vi "TranslateTyping.vi"(11 "Cluster":T2) -> (3 "string":string)   [LabVIEW 2016]
uses:
  <vilib>/event_ctls.llb/eventvkey.ctl
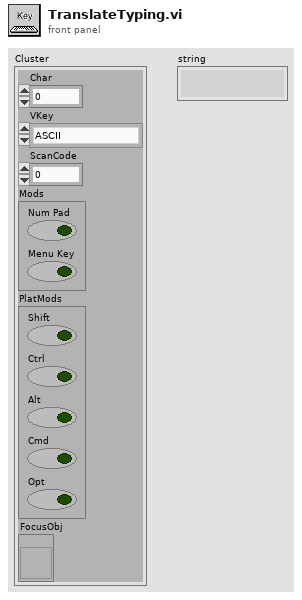
[diagram p1: front panel]
types:
  T1 = typedef "eventvkey.ctl" = enum16{"ASCII", "Enter", "Return", "Shift", "Ctrl", "Alt", "Cmd", "Opt", "Caps", "NumLock", "Clear", "Break", "Up", "Down", "Left", "Right", "Insert", "Delete", "Home", "End", "PageUp", "PageDown", "Escape", "Help", "Pause", "ScrollLock", "F1", "F2", "F3", "F4", "F5", "F6", "F7", "F8", "F9", "F10", "F11", "F12", "F13", "F14", "F15", "F16", "F17", "F18", "F19", "F20", "F21", "F22", "F23", "F24", "Play", "VolumeUp", "VolumeDown", "Mute", "Two Byte Char"}
  T2 = cluster{"Char":i16, "VKey":T1, "ScanCode":i16, "Mods":cluster{"Num Pad":bool, "Menu Key":bool}, "PlatMods":cluster{"Shift":bool, "Ctrl":bool, "Alt":bool, "Cmd":bool, "Opt":bool}, "FocusObj":refnum<vi>}
  T3 = cluster{"Shift":bool, "Ctrl":bool, "Alt":bool, "Cmd":bool, "Opt":bool}
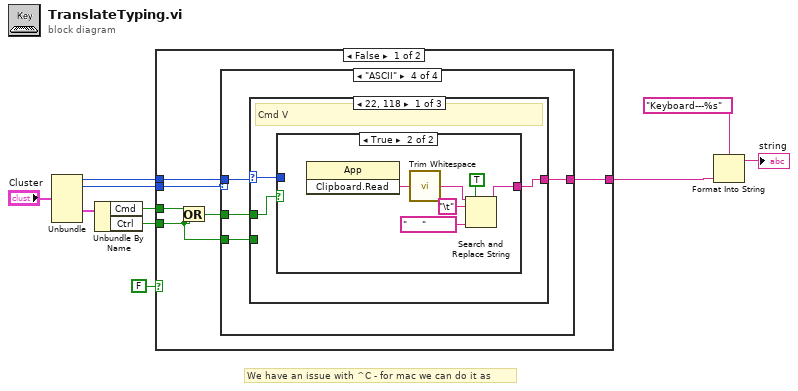
[diagram p0: block diagram]
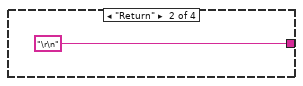
[diagram p3: hidden frame]
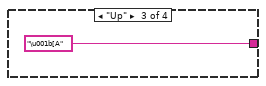
[diagram p4: hidden frame]
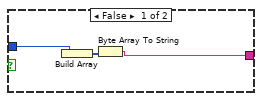
[diagram p5: hidden frame]
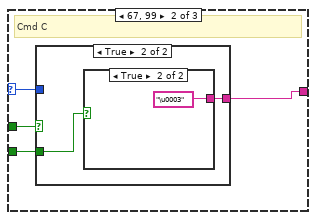
[diagram p6: hidden frame]
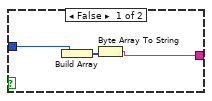
[diagram p7: hidden frame]
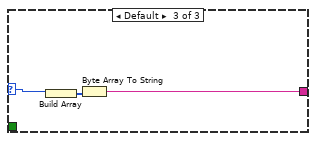
[diagram p9: hidden frame]
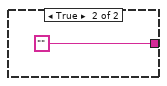
[diagram p10: hidden frame]
diagram:
  # "We have an issue with ^C - for mac we can do it as"
  n1 = Unbundle("Cluster") -> ("Char"=w9:i16, "VKey"=w8:T1, "PlatMods"=w7:T3)  [unwired: 3 out]
  n2 = Unbundle By Name(w7) -> ("Cmd"=w2:bool, "Ctrl"=w6:bool)
  n3 = case shown="False" FALSE {
    tunnel: [w16 "" ("string")] -> w5
    tunnel: w9 -> [w15 _]
    tunnel: w8 -> [w14 _]
    tunnel: w6 -> [w11 _]
    tunnel: w2 -> [w12 _]
    frame False {
      n4 = Or(x=w12, y=w11) -> (x .or. y?=w13:bool)
      n5 = case shown="\"ASCII\"" w14 {
        tunnel: [_ "\r\n" ("string") "\u001b[A" ("string") w22] -> w16
        tunnel: w15 -> [_ _ _ w21]
        tunnel: w13 -> [_ _ _ w20]
        tunnel: w11 -> [_ _ _ w19]
        frame Default {
        }
        frame "Return" {
        }
        frame "Up" {
        }
        frame "ASCII" {
          n6 = case shown="22, 118" w21 {
            selector: w21 -> [w23 w36 w45]
            tunnel: [w25 w38 w47] -> w22
            tunnel: w20 -> [w24 w37 _]
            tunnel: w19 -> [_ w35 _]
            frame 22, 118 {
              # "Cmd V"
              n7 = case shown="True" w24 {
                tunnel: [w26 w29] -> w25
                tunnel: w23 -> [w27 _]
                frame False {
                  n8 = Build Array(w27) -> (w28:i16[])
                  n9 = Byte Array To String(unsigned byte array=w28) -> (string=w26:string)
                }
                frame True {
                  n10 = invoke class="App" method="Clipboard.Read"() -> ("Read Clipbrd"=w34:string)  [unwired: 3 in, 2 out]
                  n11 = call <vilib>:"Trim Whitespace.vi"("string"=w34) -> ("trimmed string"=w33:string)  [unwired: 1 in]
                  n12 = Search and Replace String(replace all?=TRUE ("replace all? (F)"), input string=w33, search string="\t", replace string="     " ("replace string (\"\")")) -> (result string=w29:string)  [unwired: 4 in, 3 out]
                }
              }
            }
            frame 67, 99 {
              # "Cmd C"
              n13 = case shown="True" w37 {
                tunnel: [w39 w42] -> w38
                tunnel: w36 -> [w40 _]
                tunnel: w35 -> [_ w43]
                frame False {
                  n14 = Build Array(w40) -> (w41:i16[])
                  n15 = Byte Array To String(unsigned byte array=w41) -> (string=w39:string)
                }
                frame True {
                  n16 = case shown="True" w43 {
                    tunnel: [_ "\u0003"] -> w42
                    frame False {
                    }
                    frame True {
                    }
                  }
                }
              }
            }
            frame Default {
              n17 = Build Array(w45) -> (w46:i16[])
              n18 = Byte Array To String(unsigned byte array=w46) -> (string=w47:string)
            }
          }
        }
      }
    }
    frame True {
    }
  }
  n19 = Format Into String(format string="Keyboard---%s", w5) -> (resulting string=→"string":string)  [unwired: 2 in, 1 out]
